vi "lsl push chunk (NOT TESTED).vi"   [LabVIEW 2018, in "liblsl-LabVIEW.lvlib"]
uses:
  <userlib>/liblsl-LabVIEW/liblsl-LabVIEW.lvlib
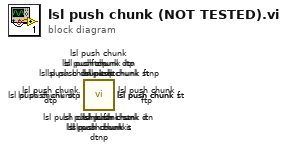
[diagram p0: block diagram]
diagram:
  n1 = call <userlib>:"lsl push chunk stn.vi"() -> ()  [unwired: 10 in, 2 out]
  n2 = call <userlib>:"lsl push chunk stnp.vi"() -> ()  [unwired: 10 in, 2 out]
  n3 = call <userlib>:"lsl push chunk stp.vi"() -> ()  [unwired: 10 in, 2 out]
  n4 = call <userlib>:"lsl push chunk st.vi"() -> ()  [unwired: 10 in, 2 out]
  n5 = call <userlib>:"lsl push chunk s.vi"() -> ()  [unwired: 10 in, 2 out]
  n6 = call <userlib>:"lsl push chunk itp.vi"() -> ()  [unwired: 10 in, 2 out]
  n7 = call <userlib>:"lsl push chunk itnp.vi"() -> ()  [unwired: 10 in, 2 out]
  n8 = call <userlib>:"lsl push chunk itn.vi"() -> ()  [unwired: 10 in, 2 out]
  n9 = call <userlib>:"lsl push chunk it.vi"() -> ()  [unwired: 10 in, 2 out]
  n10 = call <userlib>:"lsl push chunk i.vi"() -> ()  [unwired: 10 in, 2 out]
  n11 = call <userlib>:"lsl push chunk ftp.vi"() -> ()  [unwired: 10 in, 2 out]
  n12 = call <userlib>:"lsl push chunk ftnp.vi"() -> ()  [unwired: 10 in, 2 out]
  n13 = call <userlib>:"lsl push chunk ftn.vi"() -> ()  [unwired: 10 in, 2 out]
  n14 = call <userlib>:"lsl push chunk ft.vi"() -> ()  [unwired: 10 in, 2 out]
  n15 = call <userlib>:"lsl push chunk f.vi"() -> ()  [unwired: 10 in, 2 out]
  n16 = call <userlib>:"lsl push chunk dtp.vi"() -> ()  [unwired: 10 in, 2 out]
  n17 = call <userlib>:"lsl push chunk dtnp.vi"() -> ()  [unwired: 10 in, 2 out]
  n18 = call <userlib>:"lsl push chunk dtn.vi"() -> ()  [unwired: 10 in, 2 out]
  n19 = call <userlib>:"lsl push chunk dt.vi"() -> ()  [unwired: 10 in, 2 out]
  n20 = call <userlib>:"lsl push chunk d.vi"() -> ()  [unwired: 10 in, 2 out]
